vi "Init.vi"(4 "Config Hash":string, 6 "Config Version":string, 8 "error in (no error)":errorcluster, 9 "Alias (None)":string, 10 "Node Info":T1) -> (0 "error out":errorcluster, 3 "Node out":refnum<class "Node Config.lvclass">)   [LabVIEW 2020, in "VectoConfig.lvlib" / "Node Config.lvclass"]
uses:
  Node Config.lvclass
  Node Info.ctl
  Node Config.lvclass/Node Config.ctl
  VectoConfig/VectoConfig.lvlib
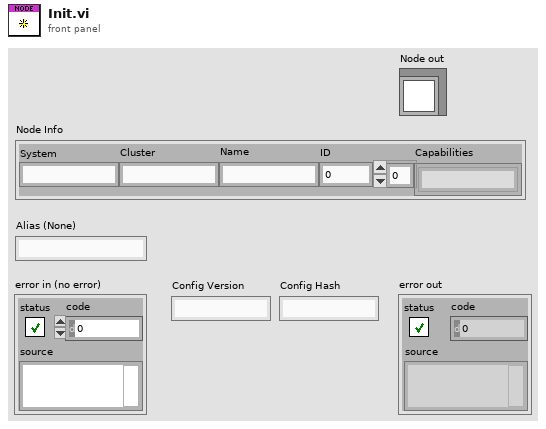
[diagram p1: front panel]
types:
  T1 = typedef "VectoConfig.lvlib/Node Info.ctl" = cluster{"System":string, "Cluster":string, "Name":string, "ID":u32, "Capabilities":string[]}
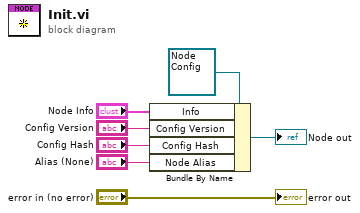
[diagram p0: block diagram]
diagram:
  n1 = Bundle By Name(cluster=refnum<class "Node Config.lvclass"> refnum ("Node in"), "Info"="Node Info", "Config Version"="Config Version", "Config Hash"="Config Hash", "Node Alias"="Alias (None)") -> (→"Node out":refnum<class "Node Config.lvclass">)
  "error out" <- "error in (no error)"
